vi "Int8 Create.vi"(8 "error in (no error)":errorcluster, 11 "I8 in":i8) -> (0 "error out":errorcluster, 3 "Int8 DVR out":refnum<data-value>)   [LabVIEW 2010, in "MDSplus.lvlib"]
uses:
  <vilib>/MDSplus/Library/MDSplus.lvlib
  <vilib>/MDSplus/Classes/Data_Class/Scalar_Class/Int8_Class/Int8.lvclass
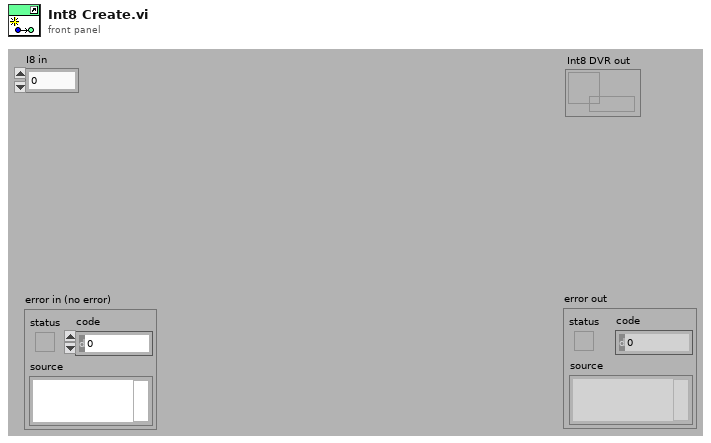
[diagram p1: front panel]
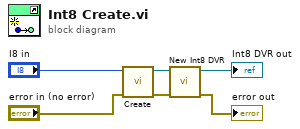
[diagram p0: block diagram]
diagram:
  n1 = call <vilib>:"Create.vi"("error in (no error)"="error in (no error)", "I8 in"="I8 in") -> ("error out"=w3:errorcluster, "Int8 out"=w4:refnum<class "Int8.lvclass">)  [unwired: 8 in]
  n2 = call <vilib>:"New Int8 DVR.vi"("error in (no error)"=w3, "Int8 in"=w4) -> ("error out"=→"error out":errorcluster, "Int8 DVR out"=→"Int8 DVR out":refnum<data-value>)  [unwired: 8 in]
